vi "Programmatically Change Tabs LV86.vi"() -> ()   [LabVIEW 2015]
panel:
  in  "stop":bool
  out "Tab Control":enum32{"Page 1", "Page 2"}(tab)
  in  "OK Button":bool
  in  "OK Button 2":bool
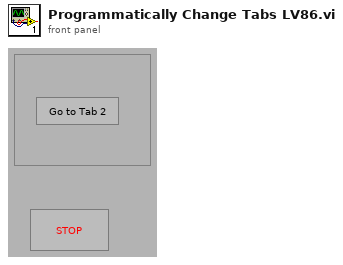
[diagram p1: front panel]
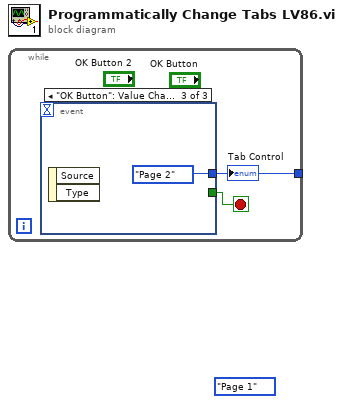
[diagram p0: block diagram]
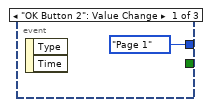
[diagram p2: hidden frame]
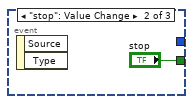
[diagram p3: hidden frame]
diagram:
  (unwired) enum32{"Page 1", "Page 2"}."Page 1" ("Tab Control")
  n1 = while {
    tunnel: [w1] -> _
    stop <- w2 stop-if-true
    n2 = event shown="[2] \"OK Button\": Value Change" {
      selector: _ -> [_ _ _]
      dyn-events: _ -> [_ _ _]
      timeout: _ -> [_ _ _]
      tunnel: [enum32{"Page 1", "Page 2"}."Page 1" ("Tab Control") _ enum32{"Page 1", "Page 2"}."Page 2" ("Tab Control")] -> w1
      tunnel: [_ "stop" _] -> w2
      event "OK Button 2": Value Change {
        n3 = event-data() -> ()  [unwired: 3 out]
      }
      event "stop": Value Change {
        n4 = event-data() -> ()  [unwired: 3 out]
      }
      event "OK Button": Value Change {
        n5 = event-data() -> ()  [unwired: 3 out]
      }
    }
    "Tab Control" <- w1
  }
